vi "SAVE_modify01.vi"() -> ()   [LabVIEW 2010]
panel:
  out "number: 0 to 1":dbl
  in  "stop":bool
  out "appended path":path
  out "System status":string
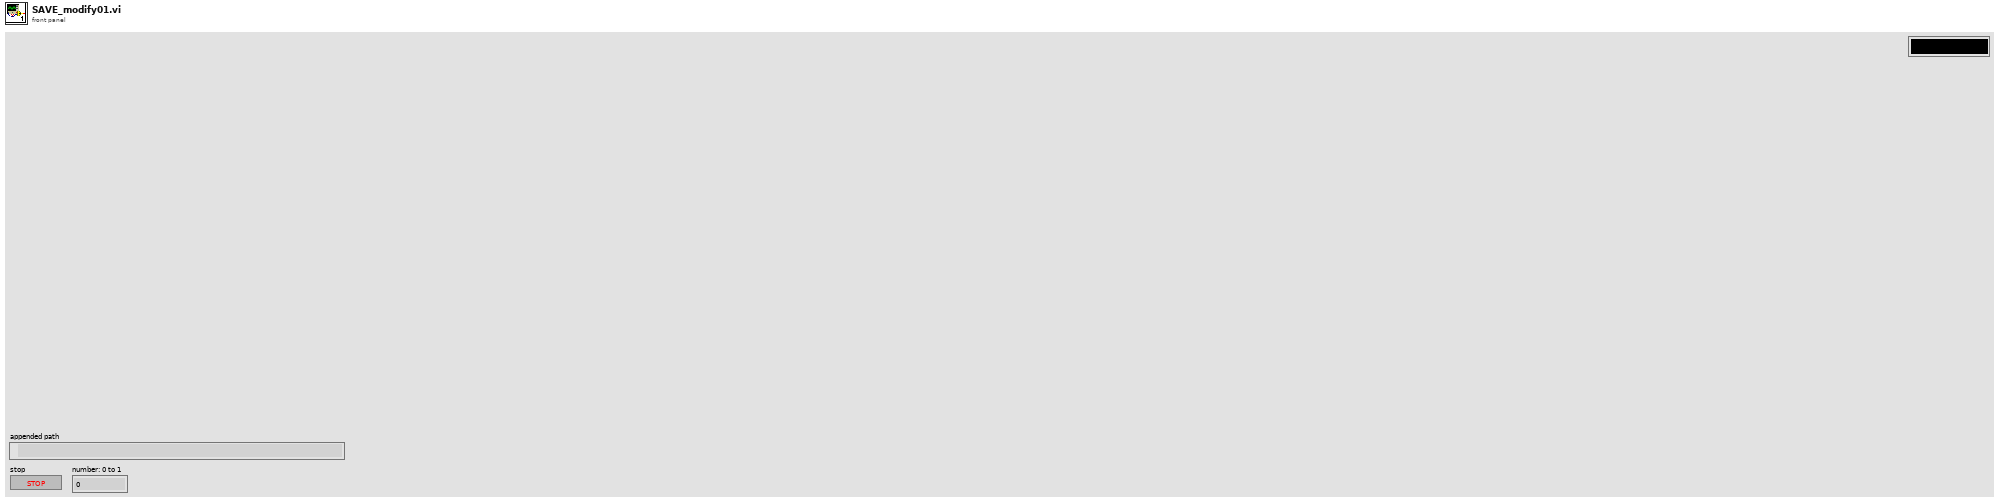
[diagram p1: front panel]
types:
  T1 = enum16{"open", "replace", "create", "open or create", "replace or create", "replace or create with confirmation"}
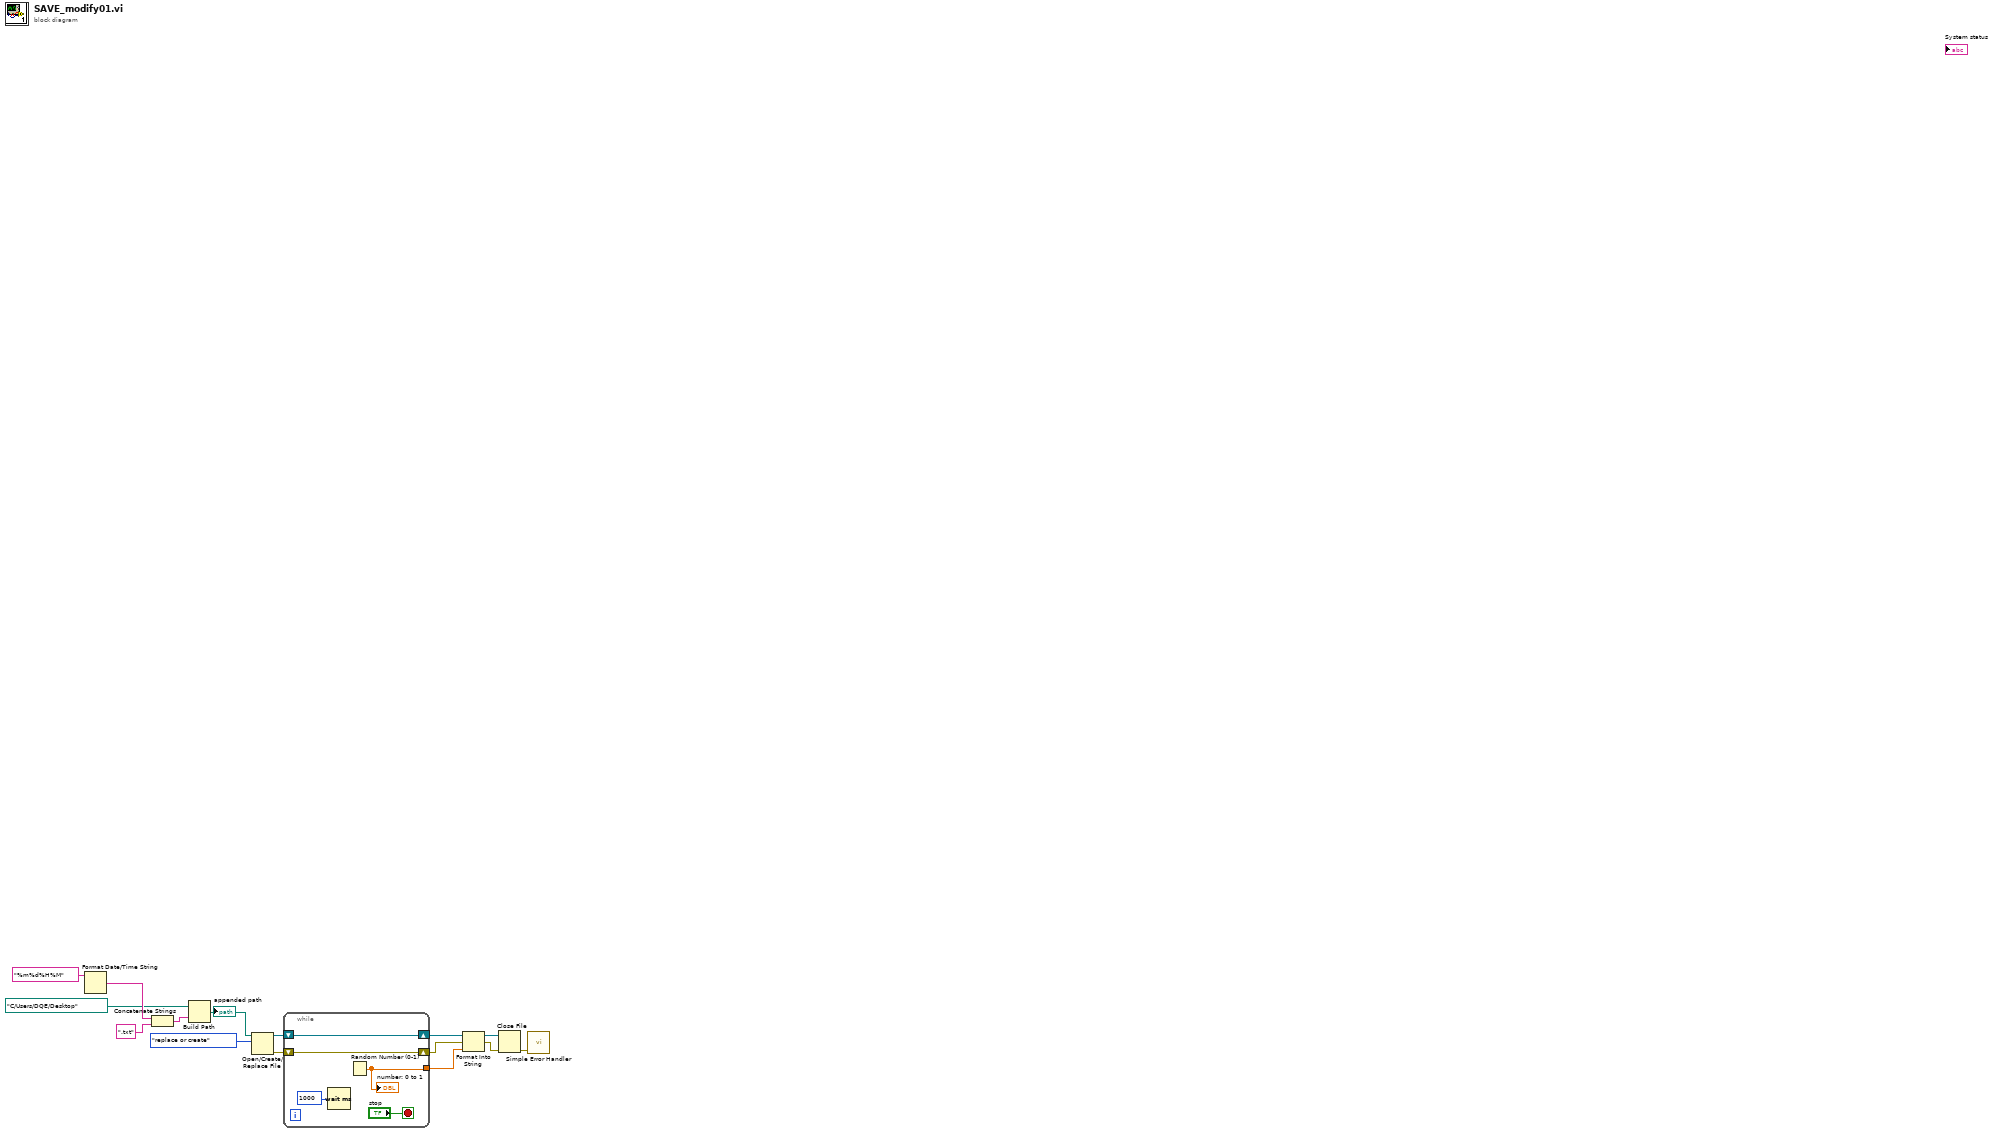
[diagram p0: block diagram]
diagram:
  n1 = Format Date/Time String(time format string (%c)="%m%d%H%M") -> (date/time string=w12:string)  [unwired: 2 in]
  n2 = Concatenate Strings(w12, ".txt" ("string")) -> (w8:string)
  n3 = Build Path(base path=path "C:/Users/DQE/Desktop", name or relative path=w8) -> (appended path=w7:path)
  "appended path" <- w7
  n4 = Open/Create/Replace File(file path (use dialog)=w7, operation (0:open)=T1."replace or create") -> (refnum out=w13:refnum<file>, error out=w14:errorcluster)  [unwired: 4 in, 1 out]
  n5 = while {
    shift-right: [w18] -> w5
    shift-left: w13 -> [w18]
    shift-right: [w17] -> w4
    shift-left: w14 -> [w17]
    tunnel: [w16] -> w1
    stop <- "stop" stop-if-true
    n6 = Wait (ms)(milliseconds to wait=u32 1000) -> ()  [unwired: 1 out]
    n7 = Random Number (0-1)() -> (number: 0 to 1=w16:dbl)
    "number: 0 to 1" <- w16
  }
  n8 = Format Into String(initial string=w5, error in=w4, w1) -> (resulting string=w3:refnum<file>, error out=w2:errorcluster)  [unwired: 1 in]
  n9 = Close File(refnum=w3, error in=w2) -> (error out=w15:errorcluster)  [unwired: 1 out]
  n10 = call <vilib>:"Simple Error Handler.vi"("error in (no error)"=w15) -> ()  [unwired: 4 in, 5 out]
